vi "Host - Update Target Data (SubVI).vi"(8 "error in":errorcluster, 10 "Addresses":string[](array[string]), 11 "Data in":T2={"VI References"=[], "Addresses"=[], "Pilot"=FALSE, "DO Data"=[], "Access Restricted?"=FALSE, "Pilot Control References"=[], "CoPilot Control References"=[], "cRIO Config"=[], "datalog Q"=refnum, "PS_P"={"AI"=[], "DI"=[], "DO"=[], "Serial"=[], "CPU"={"Total Load"=[], "Interrupt Load"=[], "Total Physical"=0.0, "Free Physical"=0.0, "Primary Disk Capacity"=0.0, "Primary Disk Free"=0.0}, "Stop"=FALSE, "DO Channel"=[]}, "PS_S"={"AI"=[], "DI"=[], "DO"=[], "Serial"=[], "CPU"={"Total Load"=[], "Interrupt Load"=[], "Total Physical"=0.0, "Free Physical"=0.0, "Primary Disk Capacity"=0.0, "Primary Disk Free"=0.0}, "Stop"=FALSE, "DO Channel"=[]}, "IDE_P"={"AI"=[], "DI"=[], "DO"=[], "Serial"=[], "CPU"={"Total Load"=[], "Interrupt Load"=[], "Total Physical"=0.0, "Free Physical"=0.0, "Primary Disk Capacity"=0.0, "Primary Disk Free"=0.0}, "Stop"=FALSE, "DO Channel"=[]}, "IDE_S"={"AI"=[], "DI"=[], "DO"=[], "Serial"=[], "CPU"={"Total Load"=[], "Interrupt Load"=[], "Total Physical"=0.0, "Free Physical"=0.0, "Primary Disk Capacity"=0.0, "Primary Disk Free"=0.0}, "Stop"=FALSE, "DO Channel"=[]}, "PDE_P"={"AI"=[], "DI"=[], "DO"=[], "Serial"=[], "CPU"={"Total Load"=[], "Interrupt Load"=[], "Total Physical"=0.0, "Free Physical"=0.0, "Primary Disk Capacity"=0.0, "Primary Disk Free"=0.0}, "Stop"=FALSE, "DO Channel"=[]}, "PDE_S"={"AI"=[], "DI"=[], "DO"=[], "Serial"=[], "CPU"={"Total Load"=[], "Interrupt Load"=[], "Total Physical"=0.0, "Free Physical"=0.0, "Primary Disk Capacity"=0.0, "Primary Disk Free"=0.0}, "Stop"=FALSE, "DO Channel"=[]}, "GUI References"={"Control Names"=[], "Control References"=[]}, "GUI Data"=[], "TCP - Serial"=[], "TCP-Serial Q"=refnum, "TCP Serial Ref"=[], "Data Sets"=[], "Last Data"=[], "Alarm Data"=[], "DI Data"=[], "Ack Data"=[], "Buzzer Data"=[], "Pilot DO"=[], "Co-Pilot DO"=[], "System Down?"=FALSE, "Log Data"=[], "Update Array"=[], "MCC Data Log"=[], "MCC Data Not"=refnum, "Thruster control"=[refnum, refnum, refnum, refnum, refnum, refnum, refnum, refnum, refnum], "waga notifier out"=refnum, "Wago  log"=[], "Thruster Cont"=[0.0, 0.0, 0.0, 0.0, 0.0, 0.0, 0.0, 0.0, 0.0], "Cam Cont"=[FALSE, FALSE, FALSE, FALSE, FALSE, TRUE], "PDE_P TH Cont"={"COM 10"=0.0, "COM 11"=0.0, "COM 12"=0.0, "COM 13"=0.0}, "PDE_S TH Cont"={"COM 10"=0.0, "COM 11"=0.0, "COM 12"=0.0, "COM 13"=0.0}} {"cRIO Config"."AI"."Interface Data"."Timing"."sample mode" items=["Finite Samples"=10178, "Continuous Samples"=10123, "Hardware Timed Single Point"=12522]; "cRIO Config"."Async"."Interface Data"."Data"."Minor Frame Count" min=5 max=8 step=1}) -> (0 "error out":errorcluster, 2 "output cluster":T1, 3 "Data out":T2={"VI References"=[], "Addresses"=[], "Pilot"=FALSE, "DO Data"=[], "Access Restricted?"=FALSE, "Pilot Control References"=[], "CoPilot Control References"=[], "cRIO Config"=[], "datalog Q"=refnum, "PS_P"={"AI"=[], "DI"=[], "DO"=[], "Serial"=[], "CPU"={"Total Load"=[], "Interrupt Load"=[], "Total Physical"=0.0, "Free Physical"=0.0, "Primary Disk Capacity"=0.0, "Primary Disk Free"=0.0}, "Stop"=FALSE, "DO Channel"=[]}, "PS_S"={"AI"=[], "DI"=[], "DO"=[], "Serial"=[], "CPU"={"Total Load"=[], "Interrupt Load"=[], "Total Physical"=0.0, "Free Physical"=0.0, "Primary Disk Capacity"=0.0, "Primary Disk Free"=0.0}, "Stop"=FALSE, "DO Channel"=[]}, "IDE_P"={"AI"=[], "DI"=[], "DO"=[], "Serial"=[], "CPU"={"Total Load"=[], "Interrupt Load"=[], "Total Physical"=0.0, "Free Physical"=0.0, "Primary Disk Capacity"=0.0, "Primary Disk Free"=0.0}, "Stop"=FALSE, "DO Channel"=[]}, "IDE_S"={"AI"=[], "DI"=[], "DO"=[], "Serial"=[], "CPU"={"Total Load"=[], "Interrupt Load"=[], "Total Physical"=0.0, "Free Physical"=0.0, "Primary Disk Capacity"=0.0, "Primary Disk Free"=0.0}, "Stop"=FALSE, "DO Channel"=[]}, "PDE_P"={"AI"=[], "DI"=[], "DO"=[], "Serial"=[], "CPU"={"Total Load"=[], "Interrupt Load"=[], "Total Physical"=0.0, "Free Physical"=0.0, "Primary Disk Capacity"=0.0, "Primary Disk Free"=0.0}, "Stop"=FALSE, "DO Channel"=[]}, "PDE_S"={"AI"=[], "DI"=[], "DO"=[], "Serial"=[], "CPU"={"Total Load"=[], "Interrupt Load"=[], "Total Physical"=0.0, "Free Physical"=0.0, "Primary Disk Capacity"=0.0, "Primary Disk Free"=0.0}, "Stop"=FALSE, "DO Channel"=[]}, "GUI References"={"Control Names"=[], "Control References"=[]}, "GUI Data"=[], "TCP - Serial"=[], "TCP-Serial Q"=refnum, "TCP Serial Ref"=[], "Data Sets"=[], "Last Data"=[], "Alarm Data"=[], "DI Data"=[], "Ack Data"=[], "Buzzer Data"=[], "Pilot DO"=[], "Co-Pilot DO"=[], "System Down?"=FALSE, "Log Data"=[], "Update Array"=[], "MCC Data Log"=[], "MCC Data Not"=refnum, "Thruster control"=[refnum, refnum, refnum, refnum, refnum, refnum, refnum, refnum, refnum], "waga notifier out"=refnum, "Wago  log"=[], "Thruster Cont"=[0.0, 0.0, 0.0, 0.0, 0.0, 0.0, 0.0, 0.0, 0.0], "Cam Cont"=[FALSE, FALSE, FALSE, FALSE, FALSE, TRUE], "PDE_P TH Cont"={"COM 10"=0.0, "COM 11"=0.0, "COM 12"=0.0, "COM 13"=0.0}, "PDE_S TH Cont"={"COM 10"=0.0, "COM 11"=0.0, "COM 12"=0.0, "COM 13"=0.0}} {"cRIO Config"."AI"."Interface Data"."Timing"."sample mode" items=["Finite Samples"=10178, "Continuous Samples"=10123, "Hardware Timed Single Point"=12522]; "cRIO Config"."Async"."Interface Data"."Data"."Minor Frame Count" min=5 max=8 step=1}, 5 "DO Change?":bool)   [LabVIEW 2021]
uses:
  Controls/Host - GUI Data Cluster.ctl
  Analog Output/Controls/AO JSON Data Cluster.ctl
  Analog Output/Controls/AO Interface Data Cluster.ctl
  Analog Output/Controls/AO Channel Configuration Cluster.ctl
  Analog Output/Controls/AO Timing Cluster.ctl
  Digital Output/Controls/DIO Configuration cluster.ctl
  Digital Output/Controls/DIO Interface Data.ctl
  Digital Output/SubVIs/Digital Dynamic Cluster.ctl
  Async JSON Cluster.ctl
  Async Interface Data Cluster.ctl
  Async Serial/Controls/Async Serial Configuration Cluster.ctl
  Async Serial/Controls/Async Frame Info Cluster.ctl
  Async Serial/Controls/Async Message Info Cluster.ctl
  Controls/Host Data Cluster.ctl
  Main Engine/Controls/Main Engine CPU Info.ctl
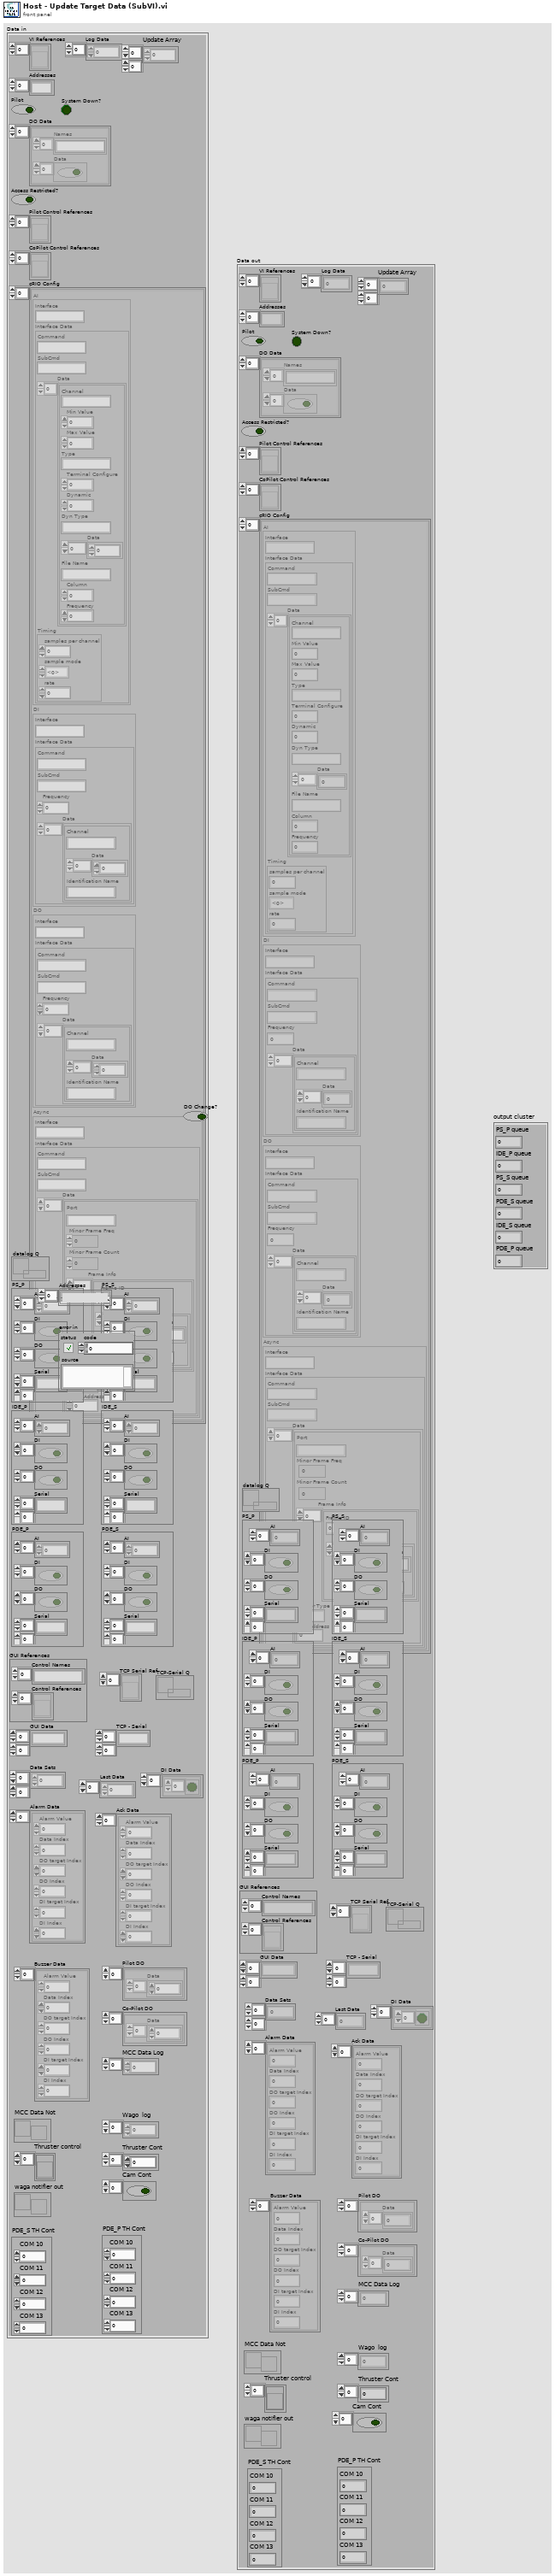
[diagram p1: front panel]
types:
  T1 = cluster{"PS_P queue":i32, "IDE_P queue":i32, "PS_S queue":i32, "PDE_S queue":i32, "IDE_S queue":i32, "PDE_P queue":i32}
  T2 = typedef "Host - GUI Data Cluster.ctl" = cluster{"VI References":refnum<vi>[], "Addresses":string[], "Pilot":bool, "DO Data":cluster{"Names":string[], "Data":bool[]}[], "Access Restricted?":bool, "Pilot Control References":refnum<vi>[], "CoPilot Control References":refnum<vi>[], "cRIO Config":cluster{"AI":T3, "DI":T7, "DO":T7, "Async":T10}[], "datalog Q":refnum<queue>, "PS_P":T15, "PS_S":T15, "IDE_P":T15, "IDE_S":T15, "PDE_P":T15, "PDE_S":T15, "GUI References":cluster{"Control Names":string[], "Control References":refnum<vi>[]}, "GUI Data":string[][], "TCP - Serial":string[][], "TCP-Serial Q":refnum<queue>, "TCP Serial Ref":refnum<vi>[], "Data Sets":dbl[][], "Last Data":dbl[], "Alarm Data":cluster{"Alarm Value":dbl, "Data Index":i32, "DO target Index":i32, "DO Index":i32, "DI target Index":i32, "DI Index":i32}[], "DI Data":cluster{bool[]}[], "Ack Data":cluster{"Alarm Value":dbl, "Data Index":i32, "DO target Index":i32, "DO Index":i32, "DI target Index":i32, "DI Index":i32}[], "Buzzer Data":cluster{"Alarm Value":dbl, "Data Index":i32, "DO target Index":i32, "DO Index":i32, "DI target Index":i32, "DI Index":i32}[], "Pilot DO":cluster{"Data":i32[]}[], "Co-Pilot DO":cluster{"Data":i32[]}[], "System Down?":bool, "Log Data":dbl[], "Update Array":i32[][], "MCC Data Log":dbl[], "MCC Data Not":refnum<notifier>, "Thruster control":refnum<vi>[], "waga notifier out":refnum<notifier>, "Wago  log":sgl[], "Thruster Cont":dbl[], "Cam Cont":bool[], "PDE_P TH Cont":cluster{"COM 10":dbl, "COM 11":dbl, "COM 12":dbl, "COM 13":dbl}, "PDE_S TH Cont":cluster{"COM 10":dbl, "COM 11":dbl, "COM 12":dbl, "COM 13":dbl}}
  T3 = typedef "AO JSON Data Cluster.ctl" = cluster{"Interface":string, "Interface Data":T4}
  T4 = typedef "AO Interface Data Cluster.ctl" = cluster{"Command":string, "SubCmd":string, "Data":T5[], "Timing":T6}
  T5 = typedef "AO Channel Configuration Cluster.ctl" = cluster{"Channel":string, "Min Value":dbl, "Max Value":dbl, "Type":string, "Terminal Configure":u16, "Dynamic":u8, "Dyn Type":string, "Data":dbl[], "File Name":string, "Column":i32, "Frequency":dbl}
  T6 = typedef "AO Timing Cluster.ctl" = cluster{"samples per channel":i32, "sample mode":i32, "rate":dbl}
  T7 = typedef "DIO Configuration cluster.ctl" = cluster{"Interface":string, "Interface Data":T8}
  T8 = typedef "DIO Interface Data.ctl" = cluster{"Command":string, "SubCmd":string, "Frequency":u16, "Data":T9[]}
  T9 = typedef "Digital Dynamic Cluster.ctl" = cluster{"Channel":string, "Data":u8[], "Identification Name":string}
  T10 = typedef "Async JSON Cluster.ctl" = cluster{"Interface":string, "Interface Data":T11}
  T11 = typedef "Async Interface Data Cluster.ctl" = cluster{"Command":string, "SubCmd":string, "Data":T12[]}
  T12 = typedef "Async Serial Configuration Cluster.ctl" = cluster{"Port":string, "Minor Frame Freq":u16, "Minor Frame Count":u16, "Frame Info":T13[], "Sensor Type":u16, "OIM Address":u16}
  T13 = typedef "Async Frame Info Cluster.ctl" = cluster{"Frame ID":u16, "Message Info":T14[]}
  T14 = typedef "Async Message Info Cluster.ctl" = cluster{"Message":u8[], "Message Name":string}
  T15 = typedef "Host Data Cluster.ctl" = cluster{"AI":dbl[], "DI":bool[], "DO":bool[], "Serial":string[][], "CPU":T16, "Stop":bool, "DO Channel":string[]}
  T16 = typedef "Main Engine CPU Info.ctl" = cluster{"Total Load":u32[], "Interrupt Load":u32[], "Total Physical":dbl, "Free Physical":dbl, "Primary Disk Capacity":dbl, "Primary Disk Free":dbl}
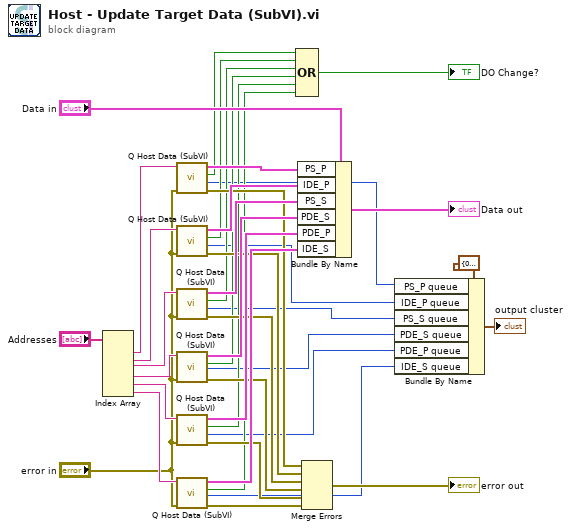
[diagram p0: block diagram]
diagram:
  n1 = Index Array(array="Addresses") -> (element #1=w16:string, element #2=w15:string, element #3=w14:string, element #4=w13:string, element #5=w12:string, element #6=w11:string)  [unwired: 6 in]
  n2 = call "Q Host Data (SubVI).vi"("error in"="error in", "IP"=w16) -> ("error out"=w29:errorcluster, "# elements in queue"=w7:i32, "DO Change?"=w22:bool, "Data"=w31:T15)  [unwired: 6 in]
  n3 = call "Q Host Data (SubVI).vi"("error in"="error in", "IP"=w15) -> ("error out"=w28:errorcluster, "# elements in queue"=w6:i32, "DO Change?"=w21:bool, "Data"=w32:T15)  [unwired: 6 in]
  n4 = call "Q Host Data (SubVI).vi"("error in"="error in", "IP"=w14) -> ("error out"=w27:errorcluster, "# elements in queue"=w5:i32, "DO Change?"=w20:bool, "Data"=w33:T15)  [unwired: 6 in]
  n5 = call "Q Host Data (SubVI).vi"("error in"="error in", "IP"=w13) -> ("error out"=w26:errorcluster, "# elements in queue"=w4:i32, "DO Change?"=w19:bool, "Data"=w34:T15)  [unwired: 6 in]
  n6 = call "Q Host Data (SubVI).vi"("error in"="error in", "IP"=w12) -> ("error out"=w25:errorcluster, "# elements in queue"=w3:i32, "DO Change?"=w18:bool, "Data"=w35:T15)  [unwired: 6 in]
  n7 = call "Q Host Data (SubVI).vi"("error in"="error in", "IP"=w11) -> ("error out"=w24:errorcluster, "# elements in queue"=w2:i32, "DO Change?"=w17:bool, "Data"=w36:T15)  [unwired: 6 in]
  n8 = Compound Arithmetic op=OR(w22, w21, w20, w19, w18, w17) -> (→"DO Change?":bool)
  n9 = Bundle By Name(cluster="Data in", "PS_P"=w31, "IDE_P"=w32, "PS_S"=w33, "PDE_S"=w34, "PDE_P"=w35, "IDE_S"=w36) -> (→"Data out":T2)
  n10 = Merge Errors(w29, w28, w27, w26, w25, w24) -> (→"error out":errorcluster)
  n11 = Bundle By Name(cluster=T1 {"PS_P queue"=0, "IDE_P queue"=0, "PS_S queue"=0, "PDE_S queue"=0, "IDE_S queue"=0, "PDE_P queue"=0}, "PS_P queue"=w7, "IDE_P queue"=w6, "PS_S queue"=w5, "PDE_S queue"=w4, "PDE_P queue"=w3, "IDE_S queue"=w2) -> (→"output cluster":T1)
